vi "FindMatchingCloseTag_NIMOD.vi"(6 "offset (0)":i32, 8 "error in":errorcluster, 9 "max offset":i32, 10 "element name":string, 11 "XML string in":string) -> (0 "error out":errorcluster, 2 "close tag":T1, 3 "content":T1, 4 "offset past close tag":i32)   [LabVIEW 2011]
doc: "This VI finds the matching XML close tagfor a given element name and returns:\n\nXML string dup - duplicate of input string\nclose tag - the contents of the close tag\noffset past match - index in string of the first character of after substring\nerror out - error output"
uses:
  Type Defs/Node Info - Cluster.ctl
panel:
  in  "error message":string="End tag not found\nfor <"
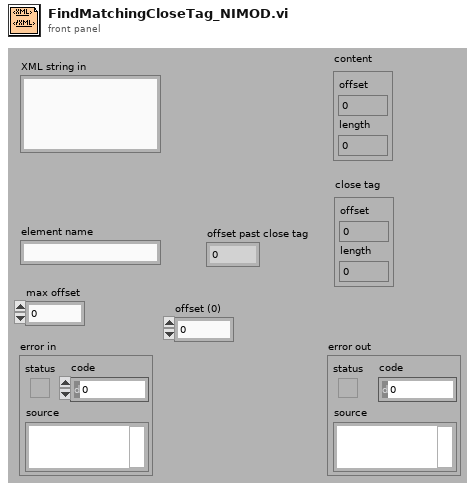
[diagram p1: front panel]
types:
  T1 = typedef "Node Info - Cluster.ctl" = cluster{"offset":i32, "length":i32}
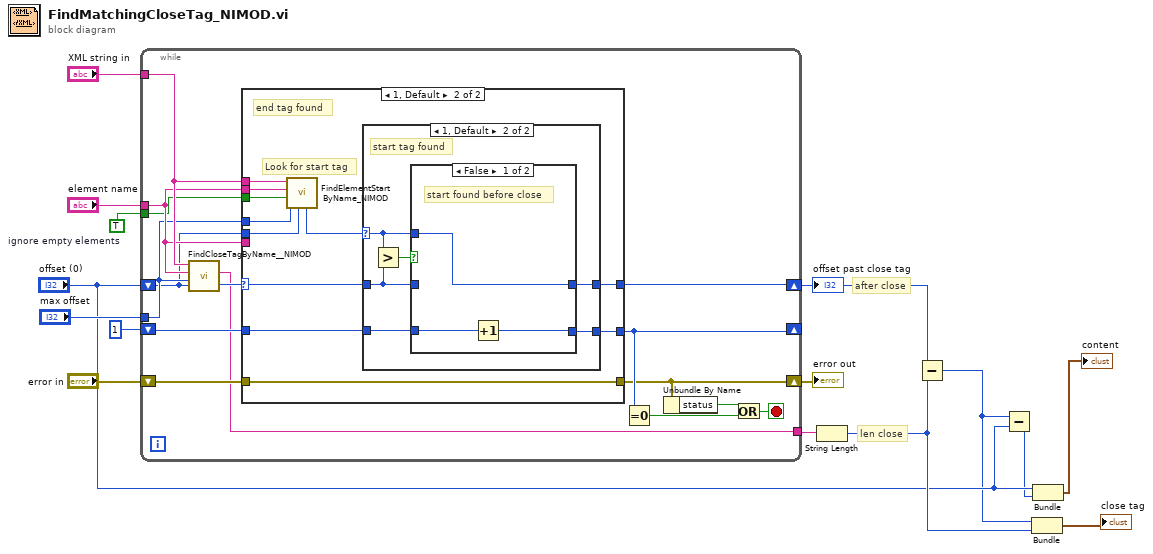
[diagram p0: block diagram]
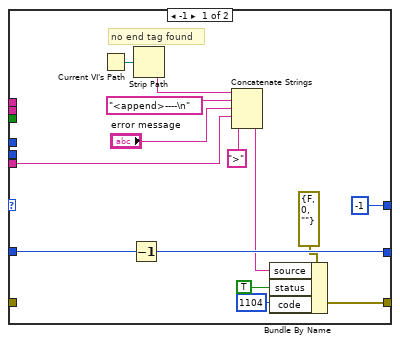
[diagram p2: hidden frame]
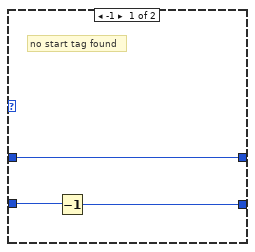
[diagram p3: hidden frame]
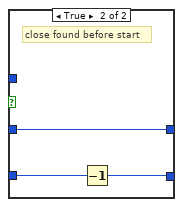
[diagram p4: hidden frame]
diagram:
  w8 = TRUE  # ignore empty elements
  # "len close"
  # "after close"
  n1 = while {
    tunnel: "XML string in" -> [w20]
    tunnel: "element name" -> [w19]
    shift-right: [w22] -> w15
    shift-left: "error in" -> [w30]
    shift-right: [w27] -> w9
    shift-left: "offset (0)" -> [w16]
    shift-right: [w25] -> _
    shift-left: 1 ("offset past match") -> [w29]
    tunnel: [w24] -> w10
    tunnel: w8 -> [w18]
    tunnel: "max offset" -> [w17]
    stop <- w23 stop-if-true
    n2 = call "FindCloseTagByName__NIMOD.vi"("offset (0)"=w16, "max offset"=w17, "close Tag"=w19, "string"=w20) -> ("match close tag"=w24:string, "offset past close tag"=w28:i32)  [unwired: 6 in]
    n3 = case shown="1, Default" w28 {
      selector: w28 -> [_ w54]
      tunnel: [-1 ("offset past match") w55] -> w27
      tunnel: w29 -> [w44 w53]
      tunnel: [w43 w52] -> w25
      tunnel: w30 -> [_ w51]
      tunnel: [w39 w51] -> w22
      tunnel: w19 -> [w32 _]
      tunnel: w20 -> [_ w50]
      tunnel: w19 -> [_ w49]
      tunnel: w18 -> [_ w48]
      tunnel: w17 -> [_ w47]
      tunnel: w16 -> [_ w46]
      frame -1 {
        # "no end tag found"
        n4 = Current VI's Path() -> (path=w37:path)
        n5 = Decrement(x=w44) -> (x-1=w43:i32)
        n6 = Strip Path(path=w37) -> (name=w36:string)  [unwired: 1 out]
        n7 = Concatenate Strings(w36, "<append>----\n" ("string"), "error message", w32, ">" ("string")) -> (w34:string)
        n8 = Bundle By Name(cluster=errorcluster {"status"=FALSE, "code"=0, "source"=""} ("error in"), "source"=w34, "status"=TRUE, "code"=1104) -> (w39:errorcluster)
      }
      frame 1, Default {
        # "Look for start tag"
        # "end tag found"
        n9 = call "FindElementStartByName_NIMOD.vi"("offset (0)"=w46, "max offset"=w47, "ignore empty elements? (false)"=w48, "Element Name"=w49, "string"=w50) -> ("offset past match"=w45:i32)  [unwired: 6 in]
        n10 = case shown="1, Default" w45 {
          selector: w45 -> [_ w59]
          tunnel: [w56 w63] -> w55
          tunnel: w54 -> [w56 w62]
          tunnel: w53 -> [w58 w61]
          tunnel: [w57 w60] -> w52
          frame -1 {
            # "no start tag found"
            n11 = Decrement(x=w58) -> (x-1=w57:i32)
          }
          frame 1, Default {
            # "start tag found"
            n12 = Greater?(x=w59, y=w62) -> (0:w64:bool)
            n13 = case shown="False" w64 {
              tunnel: w62 -> [_ w68]
              tunnel: w59 -> [w65 _]
              tunnel: [w65 w68] -> w63
              tunnel: w61 -> [w67 w70]
              tunnel: [w66 w69] -> w60
              frame False {
                # "start found before close"
                n14 = Increment(x=w67) -> (x+1=w66:i32)
              }
              frame True {
                # "close found before start"
                n15 = Decrement(x=w70) -> (x-1=w69:i32)
              }
            }
          }
        }
      }
    }
    n16 = Equal To 0?(x=w25) -> (x = 0?=w26:bool)
    n17 = Unbundle By Name(w22) -> ("status"=w21:bool)
    n18 = Or(x=w21, y=w26) -> (x .or. y?=w23:bool)
  }
  "error out" <- w15
  "offset past close tag" <- w9
  n19 = String Length(string=w10) -> (length=w5:i32)
  n20 = Subtract(x=w9, y=w5) -> (x-y=w1:i32)
  n21 = Subtract(x=w1, y="offset (0)") -> (x-y=w2:i32)
  n22 = Bundle(w1, w5) -> (→"close tag":cluster{i32, i32})  [unwired: 1 in]
  n23 = Bundle("offset (0)"="offset (0)", w2) -> (→"content":cluster{"offset (0)":i32, i32})  [unwired: 1 in]
